vi "Perform Action.vi"(8 "error in (no error)":errorcluster, 11 "Task Actor in":refnum<class "Task Actor.lvclass">) -> (0 "error out":errorcluster, 3 "Task Actor out":refnum<class "Task Actor.lvclass">)   [LabVIEW 2023, in "Task Actor.lvlib" / "Task Actor.lvclass"]
uses:
  Task Actor.lvclass
  Task Actor.lvclass/Task Actor.ctl
  Task Base/Task Base.lvclass
panel:
  out "Output":variant
  in  "Input":variant
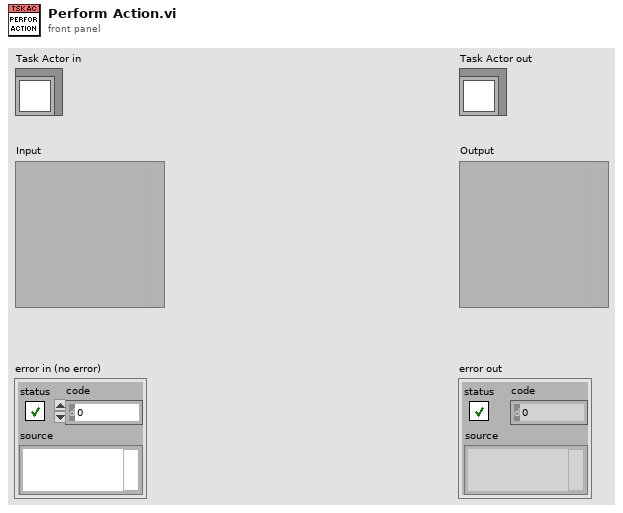
[diagram p1: front panel]
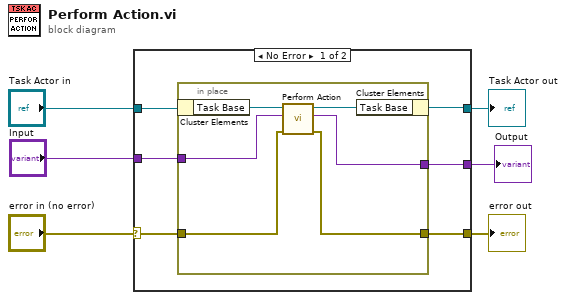
[diagram p0: block diagram]
diagram:
  n1 = case shown="No Error" "error in (no error)" {
    selector: "error in (no error)" -> [w10 w20]
    tunnel: [w9 w20] -> w5
    tunnel: [w7 w19] -> w3
    tunnel: "Task Actor in" -> [w12 w19]
    tunnel: "Input" -> [w11 _]
    tunnel: [w8 _] -> w1
    frame No Error {
      n2 = in-place {
        in-place-border: w11 -> [w17]
        in-place-border: w10 -> [w16]
        in-place-border: [w15] -> w9
        in-place-border: [w14] -> w8
        n3 = in-place-cluster #1(w12) -> ("Task Base"=w18:refnum<class "Task Base.lvclass">)
        n4 = call-dynamic "Perform Action.vi"("error in (no error)"=w16, "Input"=w17, "Task Base in"=w18) -> ("error out"=w15:errorcluster, "Output"=w14:variant, "Task Base out"=w13:refnum<class "Task Base.lvclass">)  [unwired: 6 in]
        n5 = in-place-cluster #1("Task Base"=w13) -> (w7:refnum<class "Task Actor.lvclass">)
      }
    }
    frame Error {
    }
  }
  "error out" <- w5
  "Task Actor out" <- w3
  "Output" <- w1
